vi "AppLauncher.vi"() -> ()   [LabVIEW 2016, in "Instrument.Oxford1820.lvclass"]
uses:
  Instrument.Oxford1820.lvclass
  <vilib>/JKI/JKI SMO/SMO/Typedefs/SMOState --Enum.ctl
  C:/Program Files (x86)/National Instruments/LabVIEW 2016/vi.lib/JKI/JKI SMO/SMO/SMO.lvclass
  C:/Program Files (x86)/National Instruments/LabVIEW 2016/user.lib/LevyLab/Levylab Instruments/SMOs/Instrument/Instrument.lvclass
  Instrument.Oxford1820 UI/Instrument.Oxford1820 UI.lvclass
  C:/Program Files (x86)/National Instruments/LabVIEW 2016/user.lib/LevyLab/Levylab Instruments/SMOs/Instrument UI/Instrument UI.lvclass
  C:/Program Files (x86)/National Instruments/LabVIEW 2016/vi.lib/JKI/JKI SMO/SMO.UI/SMO.UI.lvclass
  <userlib>/LevyLab/Levylab Instruments/SMOs/Instrument/Instrument.lvclass
  <vilib>/JKI/JKI SMO/SMO/SMO.lvclass
  <vilib>/JKI/JKI SMO/SMO.UI/SMO.UI.lvclass
  <vilib>/Utility/sysdir.llb/System Directory Type.ctl
  <userlib>/LevyLab/Levylab Instruments/SMOs/Instrument UI/Instrument UI.lvclass
panel:
  out "UI SMO State":T1
  out "SMO State":T1
  out "error out":errorcluster
  in  "Stop":bool
  # "Instrument.SR7270 SMO Launcher"
  # "For instructions on how to use the JKI State Machine Objects, examples and video tutorials, visit:\nhttp://jki.net/state-machine-objects/\n\nJKI State Machine Objects™\nhttp://jki.net/state-machine-objects/\nCopyright (C) 2005-2015, JKI <info@jki.net>\nALL RIGHTS RESERVED"
  # "Starting Example Instrument..."
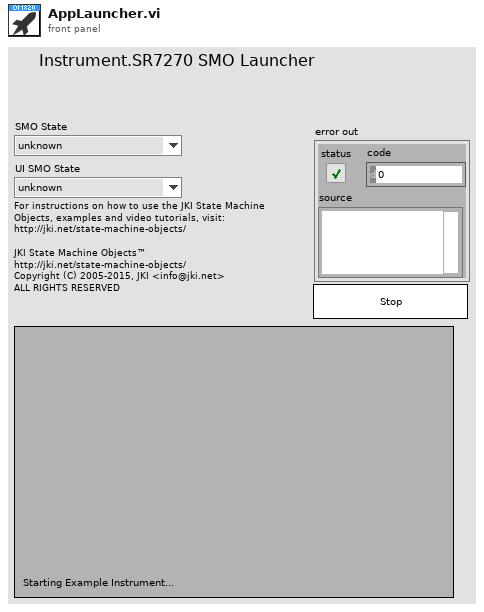
[diagram p1: front panel]
types:
  T1 = typedef "SMO.lvclass/SMOState --Enum.ctl" = enum16{"unknown", "Created", "Started", "Stopped"}
  T2 = typedef "System Directory Type.ctl" = i32
  T3 = typedef "SMO.lvclass/Public Events.ctl" = cluster{"Error":refnum<user-event>, "State":refnum<user-event>, "Reserve State":refnum<user-event>}
  T4 = cluster{"Event Registration Refnum":refnum<event-registration>, "Event Registration Refnum":refnum<event-registration>}
  T5 = enum32{"Invalid", "Standard", "Closed", "Hidden", "Minimized", "Maximized"}
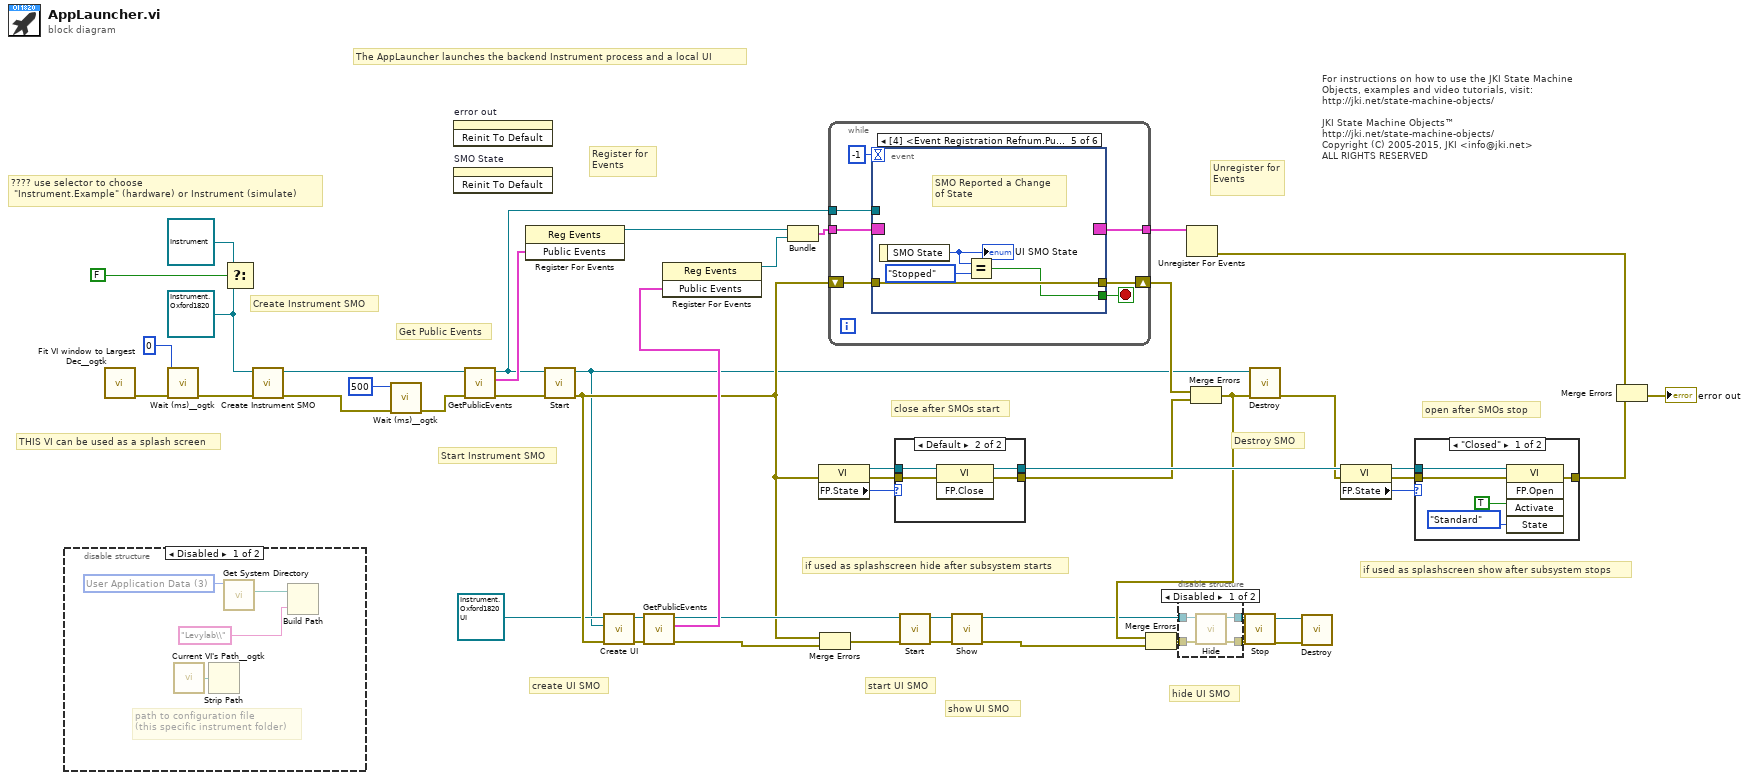
[diagram p0: block diagram]
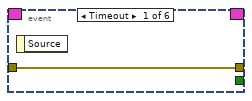
[diagram p5: hidden frame]
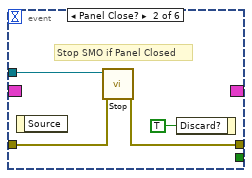
[diagram p6: hidden frame]
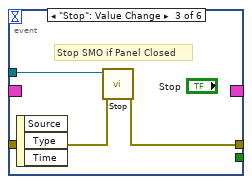
[diagram p7: hidden frame]
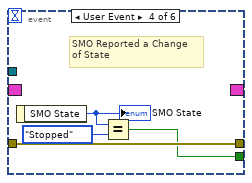
[diagram p8: hidden frame]
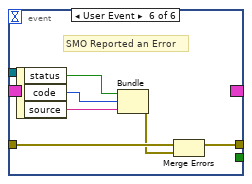
[diagram p9: hidden frame]
diagram:
  w8 = refnum<class "Instrument.Oxford1820.lvclass"> refnum ("Instrument.SR7270.lvclass")
  # "???? use selector to choose\n \"Instrument.Example\" (hardware) or Instrument (simulate)"
  # "open after SMOs stop"
  # "close after SMOs start"
  # "hide UI SMO"
  # "show UI SMO"
  # "start UI SMO"
  # "create UI SMO"
  # "if used as splashscreen show after subsystem stops"
  # "if used as splashscreen hide after subsystem starts"
  # "THIS VI can be used as a splash screen"
  # "The AppLauncher launches the backend Instrument process and a local UI"
  # "Get Public Events"
  # "Start Instrument SMO"
  # "Destroy SMO"
  # "Create Instrument SMO"
  # "Unregister for Events"
  # "Register for Events"
  # "For instructions on how to use the JKI State Machine Objects, examples and video tutorials, visit:\nhttp://jki.net/state-machine-objects/\n\nJKI State Machine Objects™\nhttp://jki.net/state-machine-objects/\nCopyright (C) 2005-2015, JKI <info@jki.net>\nALL RIGHTS RESERVED"
  n1 = disable-structure shown="Disabled" {
    frame Disabled {
      w52 = T2 3 items=["User Home"=0, "User Desktop"=1, "User Documents"=2, "User Application Data"=3, "User Preferences"=4, "User Temporary"=5, "Public Documents"=6, "Public Application Data"=7, "Public Preferences"=8, "Public Cache"=13, "System Core Libraries"=9, "System Installed Libraries"=10, "Application Files"=11, "Boot Volume Root"=12] ("system directory type")
      # "path to configuration file\n(this specific instrument folder)"
      n2 = call <userlib>:"Current VI's Path__ogtk.vi"() -> ("Current VI's Path (+ Relative)"=w53:path)  [unwired: 1 in]
      n3 = Strip Path(path=w53) -> ()  [unwired: 2 out]
      n4 = call <vilib>:"Get System Directory.vi"("system directory type"=w52) -> ("system directory"=w51:path)  [unwired: 10 in]
      n5 = Build Path(base path=w51, name or relative path="Levylab\\") -> ()  [unwired: 1 out]
    }
    frame Enabled {
    }
  }
  n6 = call <userlib>:"Fit VI window to Largest Dec__ogtk.vi"() -> ("error out"=w38:errorcluster)  [unwired: 6 in, 1 out]
  n7 = call <userlib>:"Wait (ms)__ogtk.vi"("error in (no error)"=w38, "milliseconds to wait"=u32 0) -> ("error out"=w9:errorcluster)  [unwired: 8 in, 1 out]
  n8 = Select(t=refnum<class "Instrument.lvclass"> refnum ("Instrument.lvclass"), s=FALSE, f=w8) -> ()  [unwired: 1 out]
  n9 = call-dynamic "Create Instrument SMO.vi"("error in (no error)"=w9, "Instrument in"=w8) -> ("error out"=w1:errorcluster, "Instrument out"=w2:refnum<class "Instrument.Oxford1820.lvclass">)  [unwired: 8 in]
  n10 = call <userlib>:"Wait (ms)__ogtk.vi"("error in (no error)"=w1, "milliseconds to wait"=u32 500) -> ("error out"=w12:errorcluster)  [unwired: 8 in, 1 out]
  n11 = invoke on="error out" class="Clust (strict)" method="Reinit To Default"() -> ()  [unwired: 3 in, 3 out]
  n12 = invoke on="SMO State" class="Enum (strict)" method="Reinit To Default"() -> ()  [unwired: 3 in, 3 out]
  n13 = call <vilib>:"GetPublicEvents.vi"("error in (no error)"=w12, "SMO"=w2) -> ("error out"=w44:errorcluster, "Public Events"=w46:T3, "SMO out"=w45:refnum<class "Instrument.Oxford1820.lvclass">)  [unwired: 7 in]
  n14 = register-events(w46) -> (reference out=w37:refnum<event-registration>)  [unwired: 2 in, 1 out]
  n15 = call <vilib>:"Start.vi"("error in (no error)"=w44, "SMO"=w45) -> ("error out"=w7:errorcluster, "SMO out"=w3:refnum<class "Instrument.Oxford1820.lvclass">)  [unwired: 8 in]
  n16 = call <userlib>:"Create UI.vi"("error in (no error)"=w7, "Instrument in"=w3, "Instrument UI"=refnum<class "Instrument.Oxford1820 UI.lvclass"> refnum ("SR7220 UI.lvclass")) -> ("error out"=w4:errorcluster, "Instrument UI out"=w5:refnum<class "Instrument.Oxford1820 UI.lvclass">)  [unwired: 7 in]
  n17 = call <vilib>:"GetPublicEvents.vi"("error in (no error)"=w4, "SMO"=w5) -> ("error out"=w28:errorcluster, "Public Events"=w34:T3, "SMO out"=w29:refnum<class "Instrument.Oxford1820 UI.lvclass">)  [unwired: 7 in]
  n18 = register-events(w34) -> (reference out=w35:refnum<event-registration>)  [unwired: 2 in, 1 out]
  n19 = Bundle("Event Registration Refnum"=w37, "Event Registration Refnum"=w35) -> (w36:T4)  [unwired: 1 in]
  n20 = property class="VI"(error in=w7) -> (reference out=w18:refnum<vi>, error out=w19:errorcluster, "FP.State"=w17:T5)  [unwired: 1 in]
  n21 = Merge Errors(w7, w28) -> (w33:errorcluster)
  n22 = while {
    shift-right: [w59] -> w43
    shift-left: w7 -> [w58]
    tunnel: w36 -> [w57]
    tunnel: [w56] -> w49
    tunnel: w45 -> [w55]
    stop <- w60 stop-if-true
    n23 = event shown="[4] <Event Registration Refnum.Public Events.State>: User Event" {
      selector: w57 -> [_ _ _ _ _ _]
      dyn-events: [_ _ _ _ _ _] -> w56
      timeout: -1 -> [_ _ _ _ _ _]
      tunnel: [_ _ _ w69 w73 _] -> w60
      tunnel: w55 -> [_ w65 w68 _ _ _]
      tunnel: [w61 w64 w67 w72 w76 w80] -> w59
      tunnel: w58 -> [w61 w63 w66 w72 w76 w78]
      event Timeout {
        n24 = event-data() -> ()  [unwired: 1 in, 1 out]
      }
      event Panel Close? {
        # "Stop SMO if Panel Closed"
        n25 = event-data() -> ()  [unwired: 1 in, 1 out]
        n26 = call <vilib>:"Stop.vi"("error in (no error)"=w63, "SMO"=w65) -> ("error out"=w64:errorcluster)  [unwired: 8 in, 1 out]
        n27 = event-data("Discard?"=TRUE ("OK")) -> ()  [unwired: 1 in, 1 out]
      }
      event "Stop": Value Change {
        # "Stop SMO if Panel Closed"
        n28 = event-data() -> ()  [unwired: 1 in, 3 out]
        n29 = call <vilib>:"Stop.vi"("error in (no error)"=w66, "SMO"=w68) -> ("error out"=w67:errorcluster)  [unwired: 8 in, 1 out]
      }
      event User Event {
        # "SMO Reported a Change\nof State"
        n30 = event-data() -> ("SMO State"=w71:T1)  [unwired: 1 in]
        "SMO State" <- w71
        n31 = Equal?(x=w71, y=SMOState_--Enum."Stopped") -> (x = y?=w69:bool)
      }
      event User Event {
        # "SMO Reported a Change\nof State"
        n32 = event-data() -> ("SMO State"=w75:T1)  [unwired: 1 in]
        "UI SMO State" <- w75
        n33 = Equal?(x=w75, y=SMOState_--Enum."Stopped") -> (x = y?=w73:bool)
      }
      event User Event {
        # "SMO Reported an Error"
        n34 = event-data() -> ("status"=w79:bool, "code"=w82:i32, "source"=w81:string)  [unwired: 1 in]
        n35 = Bundle("status"=w79, "code"=w82, "source"=w81) -> (w77:errorcluster)  [unwired: 1 in]
        n36 = Merge Errors(w78, w77) -> (w80:errorcluster)
      }
    }
  }
  n37 = case shown="Default" w17 {
    tunnel: [w84 w88] -> w39
    tunnel: w19 -> [w84 w87]
    tunnel: w18 -> [w83 w86]
    tunnel: [w83 w85] -> w42
    frame "Invalid", "Closed" {
    }
    frame Default {
      n38 = invoke class="VI" method="FP.Close"(reference=w86, error in=w87) -> (reference out=w85:refnum<vi>, error out=w88:errorcluster)  [unwired: 1 in, 1 out]
    }
  }
  n39 = call <vilib>:"Start.vi"("error in (no error)"=w33, "SMO"=w29) -> ("error out"=w27:errorcluster, "SMO out"=w26:refnum<class "Instrument.Oxford1820 UI.lvclass">)  [unwired: 8 in]
  n40 = call <vilib>:"Show.vi"("error in (no error)"=w27, "SMO.UI"=w26) -> ("error out"=w25:errorcluster, "SMO.UI out"=w21:refnum<class "Instrument.Oxford1820 UI.lvclass">)  [unwired: 8 in]
  n41 = Unregister For Events(event registration refnum=w49) -> (error out=w48:errorcluster)  [unwired: 1 in]
  n42 = Merge Errors(w43, w39) -> (w30:errorcluster)
  n43 = Merge Errors(w30, w25) -> (w22:errorcluster)
  n44 = disable-structure shown="Disabled" {
    disable-tunnel: [w92 w93] -> w24
    disable-tunnel: [w91 w94] -> w23
    disable-tunnel: w22 -> [w90 w93]
    disable-tunnel: w21 -> [w89 w94]
    frame Disabled {
      n45 = call <vilib>:"Hide.vi"("error in (no error)"=w90, "SMO.UI"=w89) -> ("error out"=w92:errorcluster, "SMO.UI out"=w91:refnum<class "Instrument.Oxford1820 UI.lvclass">)  [unwired: 8 in]
    }
    frame Enabled {
    }
  }
  n46 = call <vilib>:"Stop.vi"("error in (no error)"=w24, "SMO"=w23) -> ("error out"=w32:errorcluster, "SMO out"=w31:refnum<class "Instrument.Oxford1820 UI.lvclass">)  [unwired: 8 in]
  n47 = call <vilib>:"Destroy.vi"("error in (no error)"=w30, "SMO"=w3) -> ("error out"=w41:errorcluster)  [unwired: 9 in]
  n48 = call <vilib>:"Destroy.vi"("error in (no error)"=w32, "SMO"=w31) -> ()  [unwired: 9 in, 1 out]
  n49 = property class="VI"(reference=w42, error in=w41) -> (reference out=w15:refnum<vi>, error out=w16:errorcluster, "FP.State"=w14:T5)
  n50 = case shown="\"Closed\"" w14 {
    tunnel: [w97 w100] -> w40
    tunnel: w16 -> [w96 w100]
    tunnel: w15 -> [w95 _]
    frame "Closed" {
      n51 = invoke class="VI" method="FP.Open"(reference=w95, error in=w96, "Activate"=TRUE, "State"=T5."Standard") -> (error out=w97:errorcluster)  [unwired: 1 in, 4 out]
    }
    frame Default {
    }
  }
  n52 = Merge Errors(w48, w40) -> (→"error out":errorcluster)
